vi "Save Source AVI With Specified Number of Frames.vi"() -> ()   [LabVIEW 2013]
panel:
  out "Frames written":i32
  out "Codec Chosen":string
  out "Codec Names":string[](array[string])
  in  "Codec":i32=4
  in  "Save AVI Path":path=path "C:/Users/achiu/Desktop/Downloads/test_1000Frames.avi"
  in  "Source AVI File Path":path=path "C:/Users/achiu/Desktop/Downloads/test.avi"
  in  "# of frames to write":i32=1000
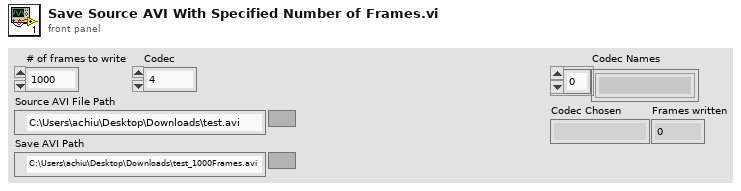
[diagram p1: front panel]
types:
  T1 = typedef "Image Type" = u32
  T2 = typedef "IMAQ AVI2 Refnum.ctl" = refnum<k20>
  T3 = typedef "IMAQ Image.ctl" = refnum<image>
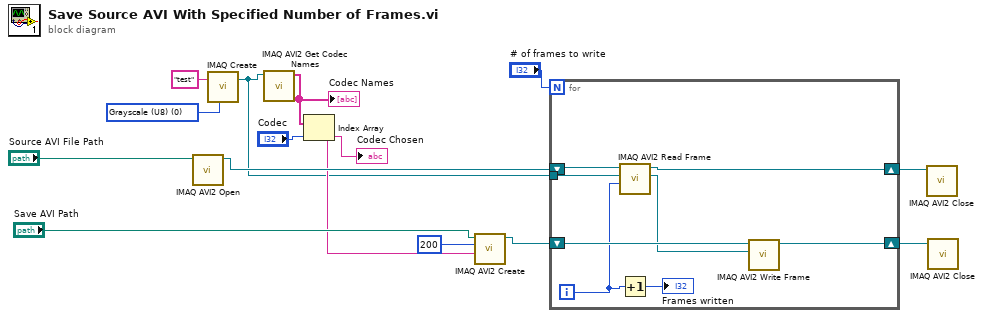
[diagram p0: block diagram]
diagram:
  w12 = T1 0 items=["Grayscale (U8)", "Grayscale (I16)", "Grayscale (SGL)", "Complex (CSG)", "RGB (U32)", "HSL (U32)", "RGB (U64)", "Grayscale (U16)"] ("Image Type")
  n1 = call "IMAQ AVI2 Open"("AVI File Path"="Source AVI File Path") -> ("AVI Refnum"=w9:T2)  [unwired: 9 in, 1 out]
  n2 = call "IMAQ Create"("Image Name"="test", "Image Type"=w12) -> ("New Image"=w4:T3)  [unwired: 3 in, 1 out]
  n3 = call "IMAQ AVI2 Get Codec Names"("Image"=w4) -> ("Codec Names"=w10:string[])  [unwired: 9 in, 1 out]
  "Codec Names" <- w10
  n4 = Index Array(array=w10, index="Codec") -> (element=w6:string)
  "Codec Chosen" <- w6
  n5 = call "IMAQ AVI2 Create"("Codec"=w6, "Frames Per Second"=u32 200, "AVI Path"="Save AVI Path") -> ("AVI Refnum"=w5:T2)  [unwired: 7 in, 1 out]
  n6 = for {
    N: "# of frames to write" -> [_]
    tunnel: w4 -> [w20]
    shift-right: [w19] -> w3
    shift-left: w9 -> [w21]
    shift-right: [w18] -> w1
    shift-left: w5 -> [w22]
    i -> [w16]
    n7 = call "IMAQ AVI2 Read Frame"("Frame Number"=w16, "Image"=w20, "AVI Refnum"=w21) -> ("Image Out"=w17:T3, "AVI Refnum (duplicate)"=w19:T2)  [unwired: 6 in, 1 out]
    n8 = Increment(x=w16) -> (x+1=→"Frames written":i32)
    n9 = call "IMAQ AVI2 Write Frame"("Image"=w17, "AVI Refnum"=w22) -> ("AVI Refnum (duplicate)"=w18:T2)  [unwired: 7 in, 2 out]
  }
  n10 = call "IMAQ AVI2 Close"("AVI Refnum"=w3) -> ()  [unwired: 10 in, 1 out]
  n11 = call "IMAQ AVI2 Close"("AVI Refnum"=w1) -> ()  [unwired: 10 in, 1 out]
